vi "Pre Launch Init.vi"(11 "Logger in":refnum<class "Logger.lvclass">) -> (0 "error out":errorcluster, 3 "Logger out":refnum<class "Logger.lvclass">)   [LabVIEW 2019, in "Logger.lvlib" / "Logger.lvclass"]
doc: "(<B>Filename</B>: Actor Framework.lvlib:Actor.lvclass:Pre Launch Init.vi)\n\nDefines behavior that occurs after the Launch Nested Actor method is invoked but before the actor's Actor Core method begins running.\n\nBy default, this method does nothing. A descendant class may override it to define behavior."
uses:
  Logger.lvclass
  Logger.lvclass/Logger.ctl
  <vilib>/ActorFramework/Actor/Actor.lvclass
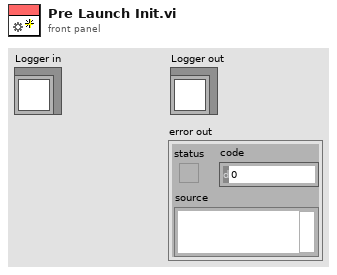
[diagram p1: front panel]
types:
  T1 = enum16{"open", "replace", "create", "open or create", "replace or create", "replace or create with confirmation"}
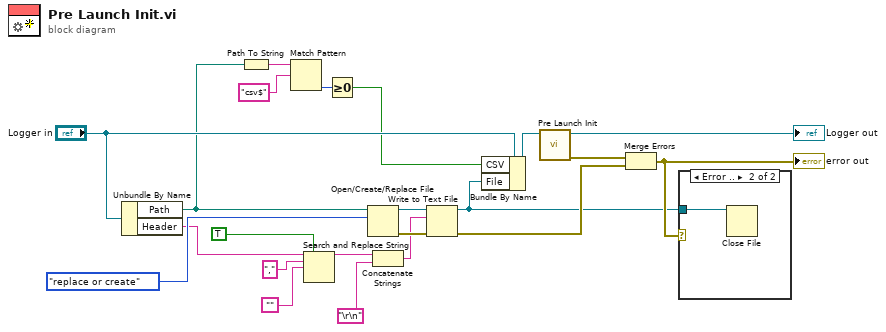
[diagram p0: block diagram]
diagram:
  n1 = Unbundle By Name("Logger in") -> ("Path"=w15:path, "Header"=w5:string)
  n2 = Path To String(path=w15) -> (string=w14:string)
  n3 = Match Pattern(string=w14, regular expression="csv$") -> (offset past match=w13:i32)  [unwired: 1 in, 3 out]
  n4 = Search and Replace String(replace all?=TRUE ("replace all? (F)"), input string=w5, search string=",", replace string="" ("replace string (\"\")")) -> (result string=w4:string)  [unwired: 4 in, 3 out]
  n5 = Greater Or Equal To 0?(x=w13) -> (x >= 0?=w12:bool)
  n6 = Open/Create/Replace File(file path (use dialog)=w15, operation (0:open)=T1."replace or create") -> (refnum out=w9:refnum<file>, error out=w17:errorcluster)  [unwired: 4 in, 1 out]
  n7 = Concatenate Strings(w4, "\r\n") -> (w6:string)
  n8 = Write to Text File(file (use dialog)=w9, text=w6, error in=w17) -> (refnum out=w8:refnum<file>, error out=w10:errorcluster)  [unwired: 1 in, 1 out]
  n9 = Bundle By Name(cluster="Logger in", "CSV"=w12, "File"=w8) -> (w18:refnum<class "Logger.lvclass">)
  n10 = call-parent "Pre Launch Init.vi"("Actor in"=w18) -> ("error out"=w22:errorcluster, "Actor out"=→"Logger out":refnum<class "Logger.lvclass">)  [unwired: 9 in]
  n11 = Merge Errors(w22, w10) -> (w16:errorcluster)
  "error out" <- w16
  n12 = case shown="Error .." w16 {
    tunnel: w8 -> [_ w23]
    frame No Error {
    }
    frame Error {
      n13 = Close File(refnum=w23) -> ()  [unwired: 1 in, 2 out]
    }
  }
